vi "TCP.IP Client for Ripple Detection_maybe4.vi"() -> ()   [LabVIEW 2021]
doc: "Demonstrates how to open a connection to an TCP server, read the data being sent, and display the data on a chart. This VI is designed to stop if the TCP connection is terminated."
uses:
  <vilib>/Analysis/3filter.llb/Butterworth Filter (DBL).vi
  <vilib>/ptbypt/NI_PtbyPt.lvlib
  <vilib>/Analysis/NI_AALBase.lvlib
panel:
  in  "File Name":path=path "F:/Career/Work/From Now/Book2.csv"
  out "Array Size 3":u32
  out "RMS2>RMS1 for 3 data":dynamicdata(graph)
  out "Array Size":u32
  in  "Boolean":bool
  in  "Server Closed":string="The server VI closed the connection."
  out "Raw Data":dbl[](graph)
  in  "Stop":bool
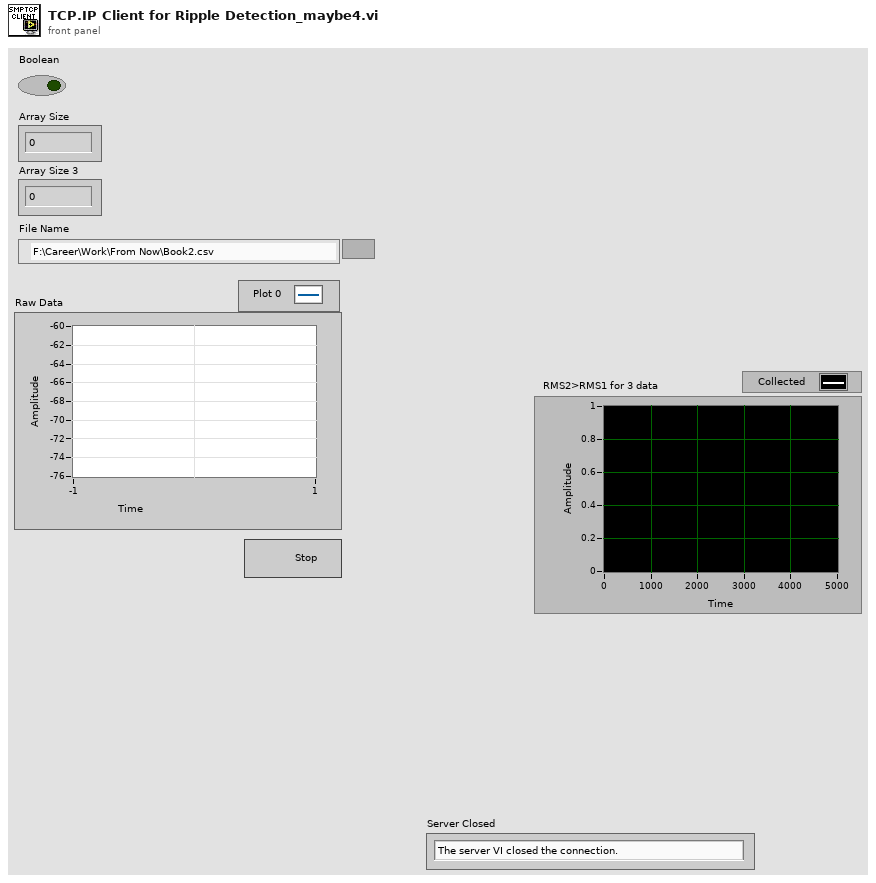
[diagram p1: front panel]
types:
  T1 = enum16{"open", "replace", "create", "open or create", "replace or create", "replace or create with confirmation"}
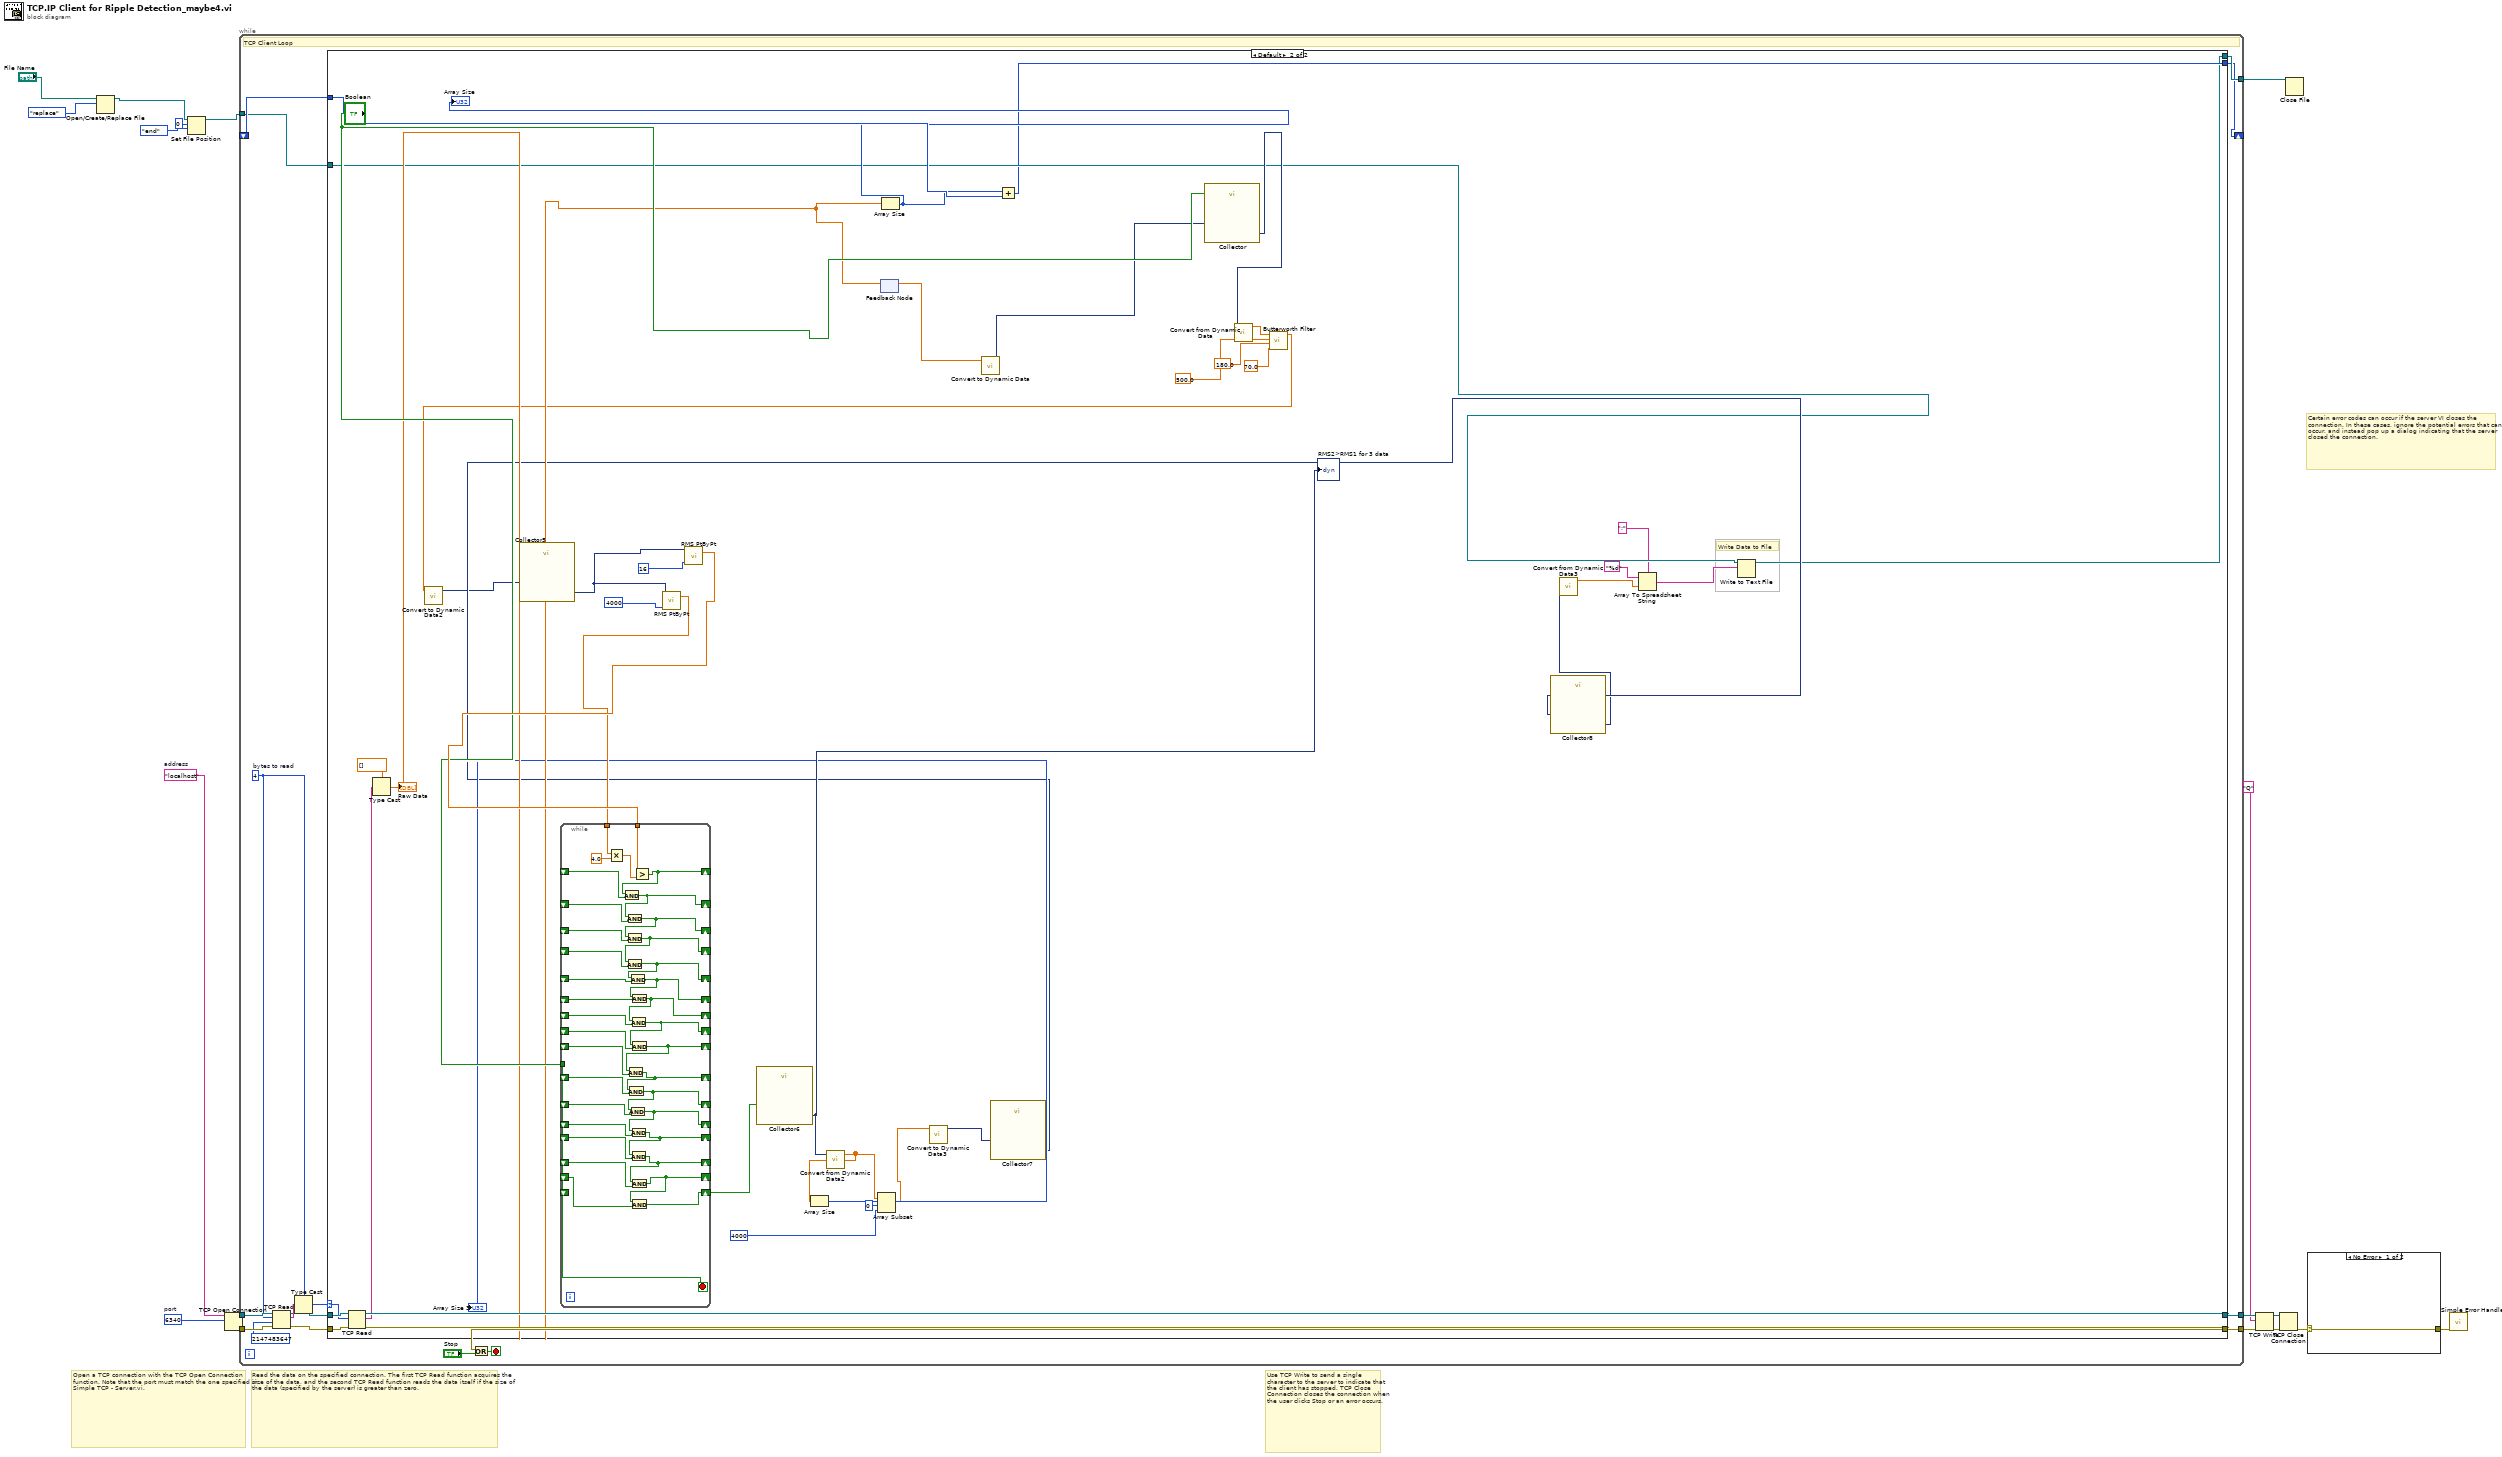
[diagram p0: block diagram]
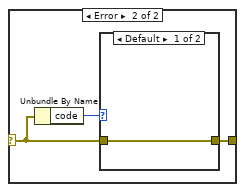
[diagram p2: hidden frame]
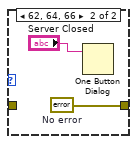
[diagram p3: hidden frame]
diagram:
  w8 = u16 6340  # port
  w9 = "localhost"  # address
  # "Certain error codes can occur if the server VI closes the connection. In these cases, ignore the potential errors that can occur, and instead pop up a dialog indicating that the server closed the connection."
  # "Use TCP Write to send a single character to the server to indicate that the client has stopped. TCP Close Connection closes the connection when the user clicks Stop or an error occurs."
  # "Read the data on the specified connection. The first TCP Read function acquires the size of the data, and the second TCP Read function reads the data itself if the size of the data (specified by the server) is greater than zero."
  # "Open a TCP connection with the TCP Open Connection function. Note that the port must match the one specified in Simple TCP - Server.vi."
  n1 = Open/Create/Replace File(file path (use dialog)="File Name", operation (0:open)=T1."replace") -> (refnum out=w2:refnum<file>)  [unwired: 4 in, 2 out]
  n2 = Set File Position(offset (in bytes) (0)=i64 0, refnum=w2, from (0:start)=enum16{"start", "end", "current"}."end") -> (refnum out=w1:refnum<file>)  [unwired: 1 in, 1 out]
  n3 = TCP Open Connection(address=w9, remote port or service name=w8) -> (connection ID=w18:refnum<k5>, error out=w17:errorcluster)  [unwired: 3 in]
  n4 = while {
    tunnel: w17 -> [w30]
    tunnel: w18 -> [w31]
    tunnel: [w26] -> w15
    tunnel: [w25] -> w13
    shift-right: [w19] -> _
    shift-left: _ -> [w22]
    tunnel: [w20] -> w7
    tunnel: w1 -> [w21]
    stop <- w27 stop-if-true
    w29 = 4  # bytes to read
    # "TCP Client Loop"
    n5 = TCP Read(connection ID=w31, bytes to read=w29, error in (no error)=w30, 9:2147483647 ("timeout ms (25000)")) -> (connection ID out=w33:refnum<k5>, data out=w34:string, error out=w32:errorcluster)  [unwired: 1 in]
    n6 = Type Cast(type=w29, x=w34) -> (*(type *) &x=w24:i32)
    n7 = case shown="Default" w24 {
      selector: w24 -> [_ w74]
      tunnel: w33 -> [w38 w80]
      tunnel: w32 -> [w37 w79]
      tunnel: [w38 w77] -> w26
      tunnel: [w37 w76] -> w25
      tunnel: w22 -> [w36 w69]
      tunnel: [w36 w40] -> w19
      tunnel: w21 -> [w35 w62]
      tunnel: [w35 w39] -> w20
      frame ..0 {
        # "The server has not written any data"
      }
      frame Default {
        # "Write Data to File"
        n8 = TCP Read(connection ID=w80, bytes to read=w74, error in (no error)=w79) -> (connection ID out=w77:refnum<k5>, data out=w75:string, error out=w76:errorcluster)  [unwired: 2 in]
        n9 = Type Cast(type=dbl[] [] ("chart"), x=w75) -> (*(type *) &x=w68:dbl[])
        "Raw Data" <- w68
        n10 = feedback #1() -> (w56:dbl[])  [unwired: 1 in]
        n11 = feedback-in #1(w68) -> ()
        n12 = Array Size(array=w68) -> (size(s)=w67:i32)
        "Array Size" <- w67
        n13 = call "Convert to Dynamic Data"("Array"=w56) -> ("Dynamic Data Type"=w57:dynamicdata)  [unwired: 3 in]
        n14 = Add(x=w67, y=w69) -> (x+y=w40:i32)
        n15 = call "Collector"("Enable"="Boolean", "Signals"=w57) -> ("Collected Signals"=w73:dynamicdata)  [unwired: 8 in, 1 out]
        n16 = call "Convert from Dynamic Data"("Dynamic Data Type"=w73) -> ("Array"=w58:dbl[])  [unwired: 3 in]
        n17 = call-poly <vilib>:"Butterworth Filter.vi"("low cutoff freq: fl"=70.0, "high cutoff freq: fh"=180.0, "sampling freq: fs"=500.0, "X"=w58) -> ("Filtered X"=w64:dbl[])  [unwired: 4 in, 1 out]
        n18 = call "Convert to Dynamic Data2"("Array"=w64) -> ("Dynamic Data Type"=w53:dynamicdata)  [unwired: 3 in]
        n19 = call "Collector5"("Signals"=w53) -> ("Collected Signals"=w52:dynamicdata)  [unwired: 9 in, 1 out]
        n20 = call <vilib>:"RMS PtByPt.vi"("sample length"=4000, "x"=w52) -> ("rms value"=w71:dbl)  [unwired: 2 in, 1 out]
        n21 = call <vilib>:"RMS PtByPt.vi"("sample length"=16, "x"=w52) -> ("rms value"=w72:dbl)  [unwired: 2 in, 1 out]
        n22 = while {
          tunnel: w72 -> [w114]
          tunnel: w71 -> [w113]
          shift-right: [w108] -> _
          shift-left: _ -> [w109]
          shift-right: [w111] -> _
          shift-left: _ -> [w110]
          tunnel: "Boolean" -> [w112]
          shift-right: [w106] -> _
          shift-left: _ -> [w107]
          shift-right: [w104] -> _
          shift-left: _ -> [w105]
          shift-right: [w103] -> _
          shift-left: _ -> [w102]
          shift-right: [w94] -> _
          shift-left: _ -> [w87]
          shift-right: [w99] -> _
          shift-left: _ -> [w98]
          shift-right: [w101] -> _
          shift-left: _ -> [w100]
          shift-right: [w96] -> _
          shift-left: _ -> [w97]
          shift-right: [w95] -> _
          shift-left: _ -> [w88]
          shift-right: [w93] -> _
          shift-left: _ -> [w86]
          shift-right: [w92] -> _
          shift-left: _ -> [w85]
          shift-right: [w91] -> _
          shift-left: _ -> [w84]
          shift-right: [w90] -> _
          shift-left: _ -> [w83]
          shift-right: [w89] -> _
          shift-left: _ -> [w82]
          shift-right: [w81] -> w46
          shift-left: _ -> [_]
          stop <- w112 stop-if-true
          n23 = Multiply(x=w113, y=4.0) -> (x*y=w115:dbl)
          n24 = Greater?(x=w114, y=w115) -> (0:w111:bool)
          n25 = And(x=w111, y=w110) -> (x .and. y?=w108:bool)
          n26 = And(x=w108, y=w109) -> (x .and. y?=w106:bool)
          n27 = And(x=w106, y=w107) -> (x .and. y?=w104:bool)
          n28 = And(x=w104, y=w105) -> (x .and. y?=w103:bool)
          n29 = And(x=w103, y=w102) -> (x .and. y?=w101:bool)
          n30 = And(x=w101, y=w100) -> (x .and. y?=w99:bool)
          n31 = And(x=w99, y=w98) -> (x .and. y?=w96:bool)
          n32 = And(x=w96, y=w97) -> (x .and. y?=w95:bool)
          n33 = And(x=w95, y=w88) -> (x .and. y?=w94:bool)
          n34 = And(x=w94, y=w87) -> (x .and. y?=w93:bool)
          n35 = And(x=w93, y=w86) -> (x .and. y?=w92:bool)
          n36 = And(x=w92, y=w85) -> (x .and. y?=w91:bool)
          n37 = And(x=w91, y=w84) -> (x .and. y?=w90:bool)
          n38 = And(x=w90, y=w83) -> (x .and. y?=w89:bool)
          n39 = And(x=w89, y=w82) -> (x .and. y?=w81:bool)
        }
        n40 = call "Collector6"("Signals"=w46) -> ("Collected Signals"=w66:dynamicdata)  [unwired: 9 in, 1 out]
        "RMS2>RMS1 for 3 data" <- w66
        n41 = call "Convert from Dynamic Data2"("Dynamic Data Type"=w66) -> ("Array"=w48:dbl[])  [unwired: 3 in]
        n42 = Array Size(array=w48) -> (size(s)=→"Array Size 3":i32)
        n43 = Array Subset(array=w48, index=0, length=4000 ("index")) -> (w47:dbl[])
        n44 = call "Convert to Dynamic Data3"("Array"=w47) -> ("Dynamic Data Type"=w51:dynamicdata)  [unwired: 3 in]
        n45 = call "Collector7"("Signals"=w51) -> ("Collected Signals"=w63:dynamicdata)  [unwired: 9 in, 1 out]
        n46 = call "Collector8"("Signals"=w63) -> ("Collected Signals"=w45:dynamicdata)  [unwired: 9 in, 1 out]
        n47 = call "Convert from Dynamic Data3"("Dynamic Data Type"=w45) -> ("Array"=w44:dbl[])  [unwired: 3 in]
        n48 = Array To Spreadsheet String(delimiter (Tab)=";" ("delimiter (\\t)"), array=w44, 3:"%d" ("format string")) -> (spreadsheet string=w43:string)
        n49 = Write to Text File(file (use dialog)=w62, text=w43) -> (refnum out=w39:refnum<file>)  [unwired: 2 in, 2 out]
      }
    }
    n50 = Or(x=w25, y="Stop") -> (x .or. y?=w27:bool)
  }
  n51 = TCP Write(connection ID=w15, data in="Q", error in (no error)=w13) -> (connection ID out=w16:refnum<k5>, error out=w14:errorcluster)  [unwired: 2 out]
  n52 = TCP Close Connection(connection ID=w16, error in (no error)=w14) -> (error out=w11:errorcluster)  [unwired: 1 in, 1 out]
  n53 = Close File(refnum=w7) -> ()  [unwired: 1 in, 2 out]
  n54 = case shown="No Error" w11 {
    selector: w11 -> [w117 w119]
    tunnel: [w117 w118] -> w10
    frame No Error {
    }
    frame Error {
      n55 = Unbundle By Name(w119) -> ("code"=w120:i32)
      n56 = case shown="Default" w120 {
        tunnel: w119 -> [w121 _]
        tunnel: [w121 w123] -> w118
        frame Default {
        }
        frame 62, 64, 66 {
          w123 = errorcluster {"status"=FALSE, "code"=0, "source"=""}  # No error
          n57 = One Button Dialog(message="Server Closed") -> ()  [unwired: 1 in, 1 out]
        }
      }
    }
  }
  n58 = call <vilib>:"Simple Error Handler.vi"("error in (no error)"=w10) -> ()  [unwired: 4 in, 5 out]
